vi "Write GenericCommClass.lvclass.vi"(8 "error in (no error)":errorcluster, 10 "StringCommClass.lvclass":refnum<class "ASCIICommClass.lvclass">, 11 "PicoMotor8742Comm in":refnum<class "PicoMotor8742Comm.lvclass">) -> (0 "error out":errorcluster, 3 "PicoMotor8742Comm out":refnum<class "PicoMotor8742Comm.lvclass">)   [LabVIEW 2020, in "PicoMotor8742Comm.lvclass"]
uses:
  PicoMotor8742Comm.lvclass
  ASCIICommClass/ASCIICommClass.lvclass
  PicoMotor8742Comm.lvclass/PicoMotor8742Comm.ctl
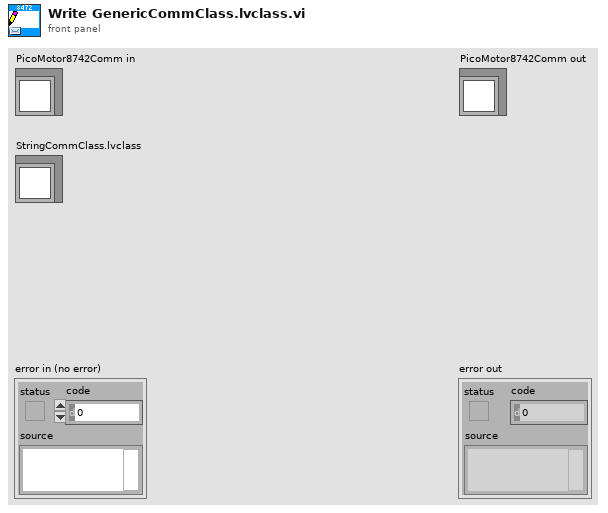
[diagram p1: front panel]
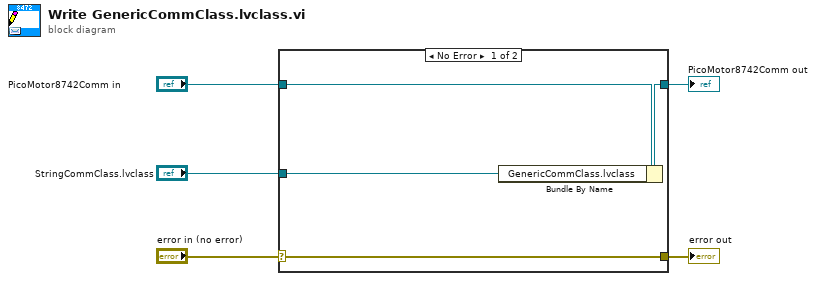
[diagram p0: block diagram]
diagram:
  n1 = case shown="No Error" "error in (no error)" {
    selector: "error in (no error)" -> [w9 w10]
    tunnel: [w9 w10] -> w4
    tunnel: [w7 w11] -> w2
    tunnel: "PicoMotor8742Comm in" -> [w8 w11]
    tunnel: "StringCommClass.lvclass" -> [w6 _]
    frame No Error {
      n2 = Bundle By Name(cluster=w8, "GenericCommClass.lvclass"=w6) -> (w7:refnum<class "PicoMotor8742Comm.lvclass">)
    }
    frame Error {
    }
  }
  "error out" <- w4
  "PicoMotor8742Comm out" <- w2
